vi "Grabber.vi"() -> ()   [LabVIEW 2014]
uses:
  <vilib>/Instr/_visa.llb/VISA Set IO Buffer Mask.ctl
  <vilib>/Instr/_visa.llb/VISA Configure Serial Port (Instr).vi
panel:
  out "GYRO_X":i16(graph)
  out "ACC_Z":i16(graph)
  in  "stop":bool
  in  "VISA resource name":refnum<visa-resource-name>
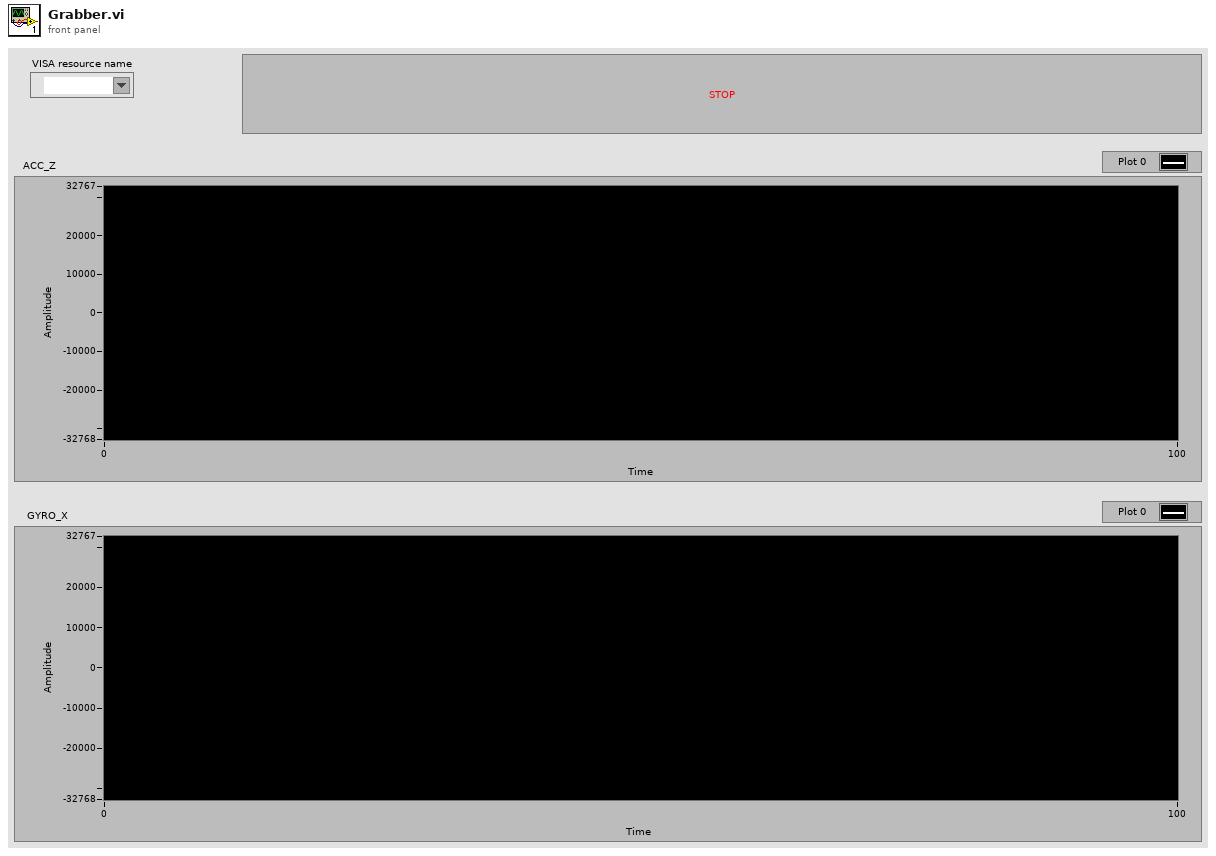
[diagram p1: front panel]
types:
  T1 = typedef "VISA Set IO Buffer Mask.ctl" = u16
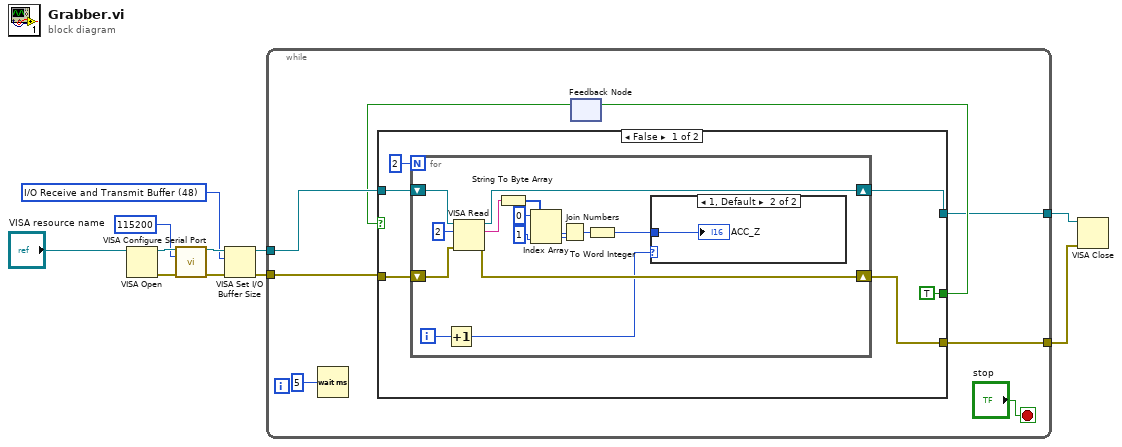
[diagram p0: block diagram]
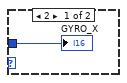
[diagram p2: hidden frame]
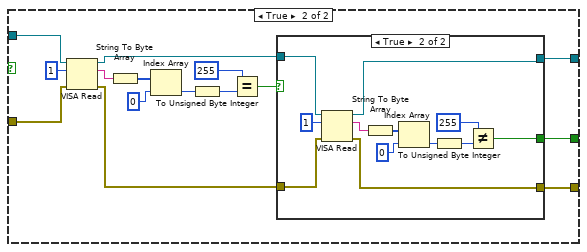
[diagram p3: hidden frame]
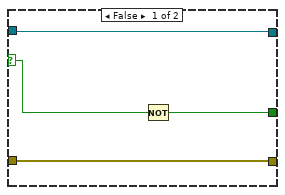
[diagram p4: hidden frame]
diagram:
  w7 = T1 48 items=["I/O Receive Buffer"=16, "I/O Transmit Buffer"=32, "I/O Receive and Transmit Buffer"=48] ("Mask")
  n1 = VISA Open(VISA resource name="VISA resource name") -> (VISA resource name=w11:refnum<visa-resource-name>, error out=w8:errorcluster)  [unwired: 4 in]
  n2 = call-poly "VISA Configure Serial Port"("VISA resource name"=w11, "baud rate (9600)"=u32 115200, "error in (no error)"=w8) -> ("VISA resource name out"=w10:refnum<visa-resource-name>, "error out"=w9:errorcluster)  [unwired: 11 in]
  n3 = VISA Set I/O Buffer Size(VISA resource name=w10, mask (16)=w7, error in (no error)=w9) -> (VISA resource name out=w5:refnum<visa-resource-name>, error out=w4:errorcluster)  [unwired: 1 in]
  n4 = while {
    tunnel: w5 -> [w18]
    tunnel: w4 -> [w17]
    tunnel: [w14] -> w2
    tunnel: [w13] -> w1
    stop <- "stop" stop-if-true
    n5 = Wait (ms)(milliseconds to wait=u32 5) -> ()  [unwired: 1 out]
    n6 = feedback #1() -> (w15:bool)  [unwired: 1 in]
    n7 = case shown="False" w15 {
      tunnel: w18 -> [w20 w57]
      tunnel: w17 -> [w25 w56]
      tunnel: [w24 w45] -> w13
      tunnel: [w23 w47] -> w14
      tunnel: [TRUE w43] -> w16
      frame False {
        n8 = for {
          N: 2 -> [_]
          shift-right: [w35] -> w23
          shift-left: w20 -> [w38]
          shift-right: [w36] -> w24
          shift-left: w25 -> [w37]
          i -> [w27]
          n9 = Increment(x=w27) -> (x+1=w26:i32)
          n10 = VISA Read(VISA resource name=w38, byte count=u32 2, error in (no error)=w37) -> (VISA resource name out=w35:refnum<visa-resource-name>, read buffer=w39:string, error out=w36:errorcluster)  [unwired: 1 out]
          n11 = String To Byte Array(string=w39) -> (unsigned byte array=w34:u8[])
          n12 = Index Array(array=w34, index #1=0 ("index"), index #2=1 ("index")) -> (element #1=w31:u8, element #2=w30:u8)
          n13 = Join Numbers(hi=w31, lo=w30) -> ((hi.lo)=w29:u16)
          n14 = To Word Integer(number=w29) -> (16bit integer=w28:i16)
          n15 = case shown="1, Default" w26 {
            tunnel: w28 -> [w41 w42]
            frame 2 {
              "GYRO_X" <- w41
            }
            frame 1, Default {
              "ACC_Z" <- w42
            }
          }
        }
      }
      frame True {
        n16 = VISA Read(VISA resource name=w57, byte count=u32 1, error in (no error)=w56) -> (VISA resource name out=w48:refnum<visa-resource-name>, read buffer=w51:string, error out=w46:errorcluster)  [unwired: 1 out]
        n17 = String To Byte Array(string=w51) -> (unsigned byte array=w54:u8[])
        n18 = Index Array(array=w54, index=0) -> (element=w52:u8)
        n19 = To Unsigned Byte Integer(number=w52) -> (unsigned 8bit integer=w49:u8)
        n20 = Equal?(x=u8 255, y=w49) -> (x = y?=w44:bool)
        n21 = case shown="True" w44 {
          selector: w44 -> [w59 _]
          tunnel: w48 -> [w60 w66]
          tunnel: [w60 w65] -> w47
          tunnel: w46 -> [w61 w64]
          tunnel: [w61 w63] -> w45
          tunnel: [w58 w62] -> w43
          frame False {
            n22 = Not(x=w59) -> (.not. x?=w58:bool)
          }
          frame True {
            n23 = VISA Read(VISA resource name=w66, byte count=u32 1, error in (no error)=w64) -> (VISA resource name out=w65:refnum<visa-resource-name>, read buffer=w69:string, error out=w63:errorcluster)  [unwired: 1 out]
            n24 = String To Byte Array(string=w69) -> (unsigned byte array=w72:u8[])
            n25 = Index Array(array=w72, index=0) -> (element=w70:u8)
            n26 = To Unsigned Byte Integer(number=w70) -> (unsigned 8bit integer=w67:u8)
            n27 = Not Equal?(x=u8 255, y=w67) -> (x != y?=w62:bool)
          }
        }
      }
    }
    n28 = feedback-in #1(w16) -> ()
  }
  n29 = VISA Close(VISA resource name=w2, error in (no error)=w1) -> ()  [unwired: 1 out]
